vi "Pure Pursuit.vi"(0 "Lookahead":dbl, 1 "Trackwidth":dbl=30.0 format="%#_13g", 2 "kffv":dbl, 3 "kffa":dbl, 5 "Odometry":T1, 7 "Max Velocity":dbl, 9 "Max Accel":dbl, 11 "error in (no error)":errorcluster) -> (4 "Left Velocity":dbl, 6 "Right Velocity":dbl, 8 "Target Point":T5, 10 "Close Point":T5, 12 "Finished?":bool, 13 "index out":i32, 14 "Curvature":dbl, 15 "error out":errorcluster)   [LabVIEW 2019, in "Pure Pursuit.lvlib"]
uses:
  Pure Pursuit.lvlib
  Typedef/Path Point.ctl
  Odometry/Typedef/Odometry.ctl
  <vilib>/Rock Robotics/WPI/ThirdParty/WPILib Extensions/Geometry/Typedef/Pose2d.ctl
  <vilib>/Rock Robotics/WPI/ThirdParty/WPILib Extensions/Geometry/Typedef/Translation2d.ctl
  <vilib>/Rock Robotics/WPI/ThirdParty/WPILib Extensions/Geometry/Typedef/Rotation2d.ctl
  Odometry/Typedef/Velocity Data.ctl
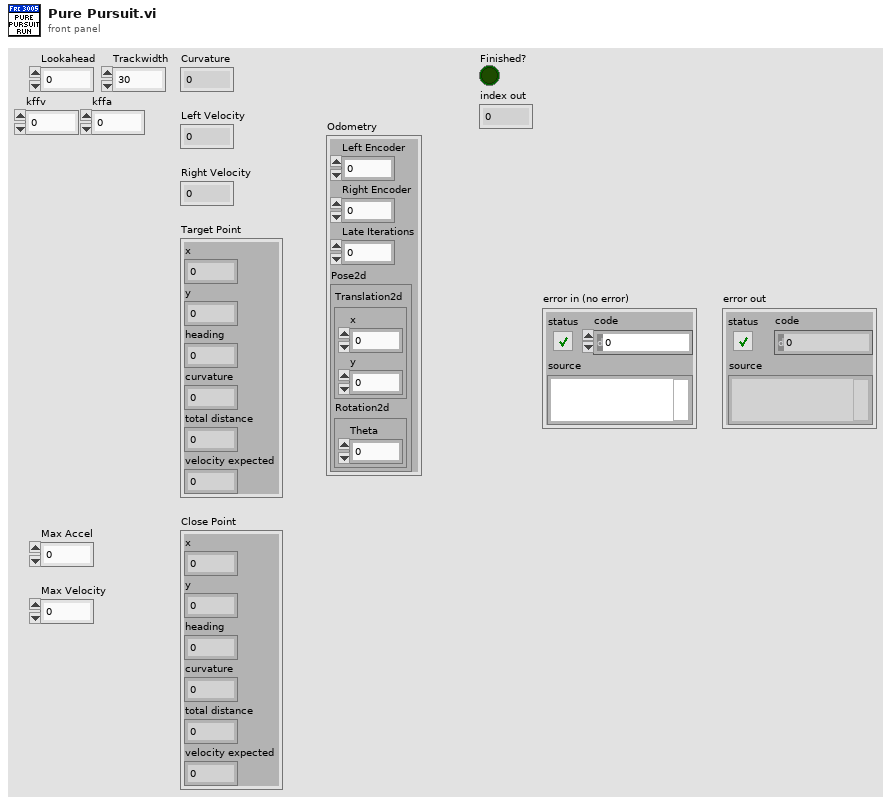
[diagram p1: front panel]
types:
  T1 = typedef "Odometry.ctl" = cluster{"Left Encoder":dbl, "Right Encoder":dbl, "Late Iterations":u32, "Pose2d":T2}
  T2 = typedef "Pose2d.ctl" = cluster{"Translation2d":T3, "Rotation2d":T4}
  T3 = typedef "Translation2d.ctl" = cluster{"x":dbl, "y":dbl}
  T4 = typedef "Rotation2d.ctl" = cluster{"Theta":dbl}
  T5 = typedef "Pure Pursuit.lvlib/Path Point.ctl" = cluster{"x":dbl, "y":dbl, "heading":dbl, "curvature":dbl, "total distance":dbl, "velocity expected":dbl}
  T6 = typedef "Velocity Data.ctl" = cluster{"Right Velocity Raw":sgl, "Left Velocity Raw":sgl, "Left Setpoint":dbl, "Right Setpoint":dbl}
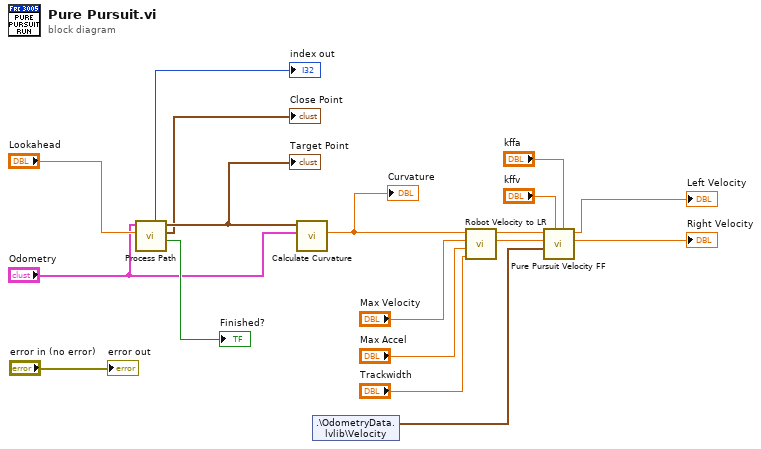
[diagram p0: block diagram]
diagram:
  n1 = call "Process Path.vi"("Lookahead"="Lookahead", "Odometry"="Odometry") -> ("Finished?"=→"Finished?":bool, "Close Point"=→"Close Point":T5, "Target Point"=w17:T5, "index out"=→"index out":i32)  [unwired: 6 in]
  "Target Point" <- w17
  n2 = call "Calculate Curvature.vi"("Odometry"="Odometry", "Target Point"=w17) -> ("Curvature"=w16:dbl)  [unwired: 8 in, 1 out]
  "Curvature" <- w16
  n3 = shared-variable ".\\OdometryData.lvlib\\Velocity"() -> (w1:T6)  [unwired: 1 in, 1 out]
  n4 = call "Robot Velocity to LR.vi"("Trackwidth"="Trackwidth", "Max Accel"="Max Accel", "Max Velocity"="Max Velocity", "Curvature"=w16) -> ("r"=w8:dbl, "l"=w9:dbl)  [unwired: 6 in]
  n5 = call "Pure Pursuit Velocity FF.vi"("kffa"="kffa", "kffv"="kffv", "Velocity"=w1, "Right Desired Velocity"=w8, "Left Desired Velocity"=w9) -> ("Right Velocity"=→"Right Velocity":dbl, "Left Velocity"=→"Left Velocity":dbl)  [unwired: 5 in]
  "error out" <- "error in (no error)"
